vi "Get VI Probes.vi"(8 "error in":errorcluster, 11 "VI Reference in":refnum<vi>) -> (0 "error out":errorcluster, 2 "Probes":i32[](array[numeric]), 3 "VI Reference out":refnum<vi>)   [LabVIEW 2020]
doc: "This VI retrieves the <b>UIDs</b> of all wires that have probes in the active VI."
uses:
  <vilib>/Utility/traverseref.llb/TRef TravTarget.ctl
  Type Definitions/Class Name--enum.ctl
  <vilib>/Utility/traverseref.llb/VI Scripting - Traverse.lvlib
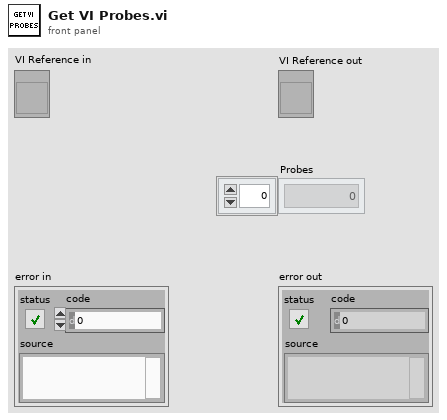
[diagram p1: front panel]
types:
  T1 = typedef "Class Name--enum.ctl" = enum16{"Node", "Wire"}
  T2 = typedef "TRef TravTarget.ctl" = enum16{"FP", "BD", "Other"}
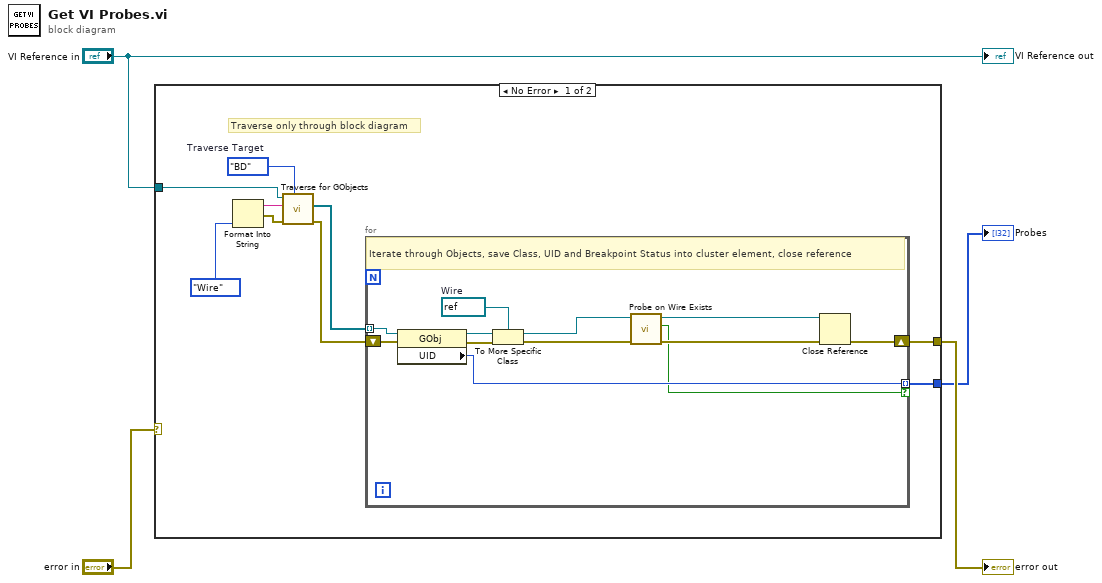
[diagram p0: block diagram]
diagram:
  n1 = case shown="No Error" "error in" {
    selector: "error in" -> [_ w26]
    tunnel: "VI Reference in" -> [w10 _]
    tunnel: [w11 w26] -> w3
    tunnel: [w6 _] -> w2
    frame No Error {
      w9 = TRef_TravTarget."BD"  # Traverse Target
      # "Traverse only through block diagram"
      n2 = Format Into String(Class_Name--enum."Wire" ("Class Name")) -> (resulting string=w7:string, error out=w12:errorcluster)  [unwired: 3 in]
      n3 = call <vilib>:"Traverse for GObjects.vi"("Traverse Target"=w9, "error in (no error)"=w12, "Class Name"=w7, "VI Refnum"=w10) -> ("error out"=w13:errorcluster, "References"=w8:refnum<vi>[])  [unwired: 4 in, 2 out]
      n4 = for {
        tunnel: w8 -> [w20] mode=indexing
        shift-right: [w23] -> w11
        shift-left: w13 -> [w25]
        tunnel: [w15] -> w6 mode=indexing if=w14
        w17 = refnum<vi> refnum  # Wire
        # "Iterate through Objects, save Class, UID and Breakpoint Status into cluster element, close reference"
        n5 = property class="GObj"(reference=w20, error in=w25) -> (reference out=w19:refnum<vi>, error out=w24:errorcluster, "UID"=w15:i32)
        n6 = To More Specific Class(target class=w17, reference=w19, error in=w24) -> (specific class reference=w16:refnum<vi>, error out=w22:errorcluster)
        n7 = call "Probe on Wire Exists.vi"("error in"=w22, "Wire in"=w16) -> ("error out"=w21:errorcluster, "Probe Exists"=w14:bool, "Wire out"=w18:refnum<vi>)  [unwired: 6 in, 1 out]
        n8 = Close Reference(reference=w18, error in (no error)=w21) -> (error out=w23:errorcluster)
      }
    }
    frame Error {
      # "Pass error without further action"
    }
  }
  "error out" <- w3
  "Probes" <- w2
  "VI Reference out" <- "VI Reference in"
